vi "Termómetro.vi"(3 "Temp Scale":bool) -> (1 "Thermometer":dbl(slide) scale=0.0..100.0)   [LabVIEW 2018]
panel:
  # "Deg C"
  # "Deg F"
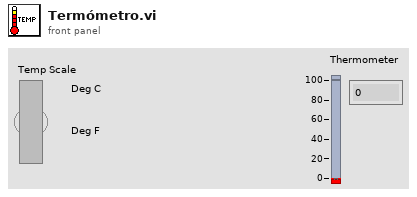
[diagram p1: front panel]
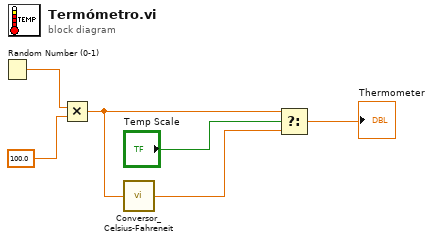
[diagram p0: block diagram]
diagram:
  n1 = Random Number (0-1)() -> (number: 0 to 1=w5:dbl)
  n2 = Multiply(x=w5, y=100.0) -> (x*y=w1:dbl)
  n3 = call "Conversor_Celsius-Fahreneit.vi"("Deg C"=w1) -> ("Deg F"=w2:dbl)
  n4 = Select(t=w1, s="Temp Scale", f=w2) -> (s? t:f=→"Thermometer":dbl)
